vi "Read Instrument ID.vi"(8 "error in (no error)":errorcluster, 11 "Generic Instrument in":refnum<class "Generic Instrument.lvclass">) -> (0 "error out":errorcluster, 2 "Instrument ID":string, 3 "Generic Instrument out":refnum<class "Generic Instrument.lvclass">)   [LabVIEW 2014, in "Generic Instrument.lvlib" / "Generic Instrument.lvclass"]
uses:
  Generic Instrument.lvclass
  Generic Instrument.lvclass/Generic Instrument.ctl
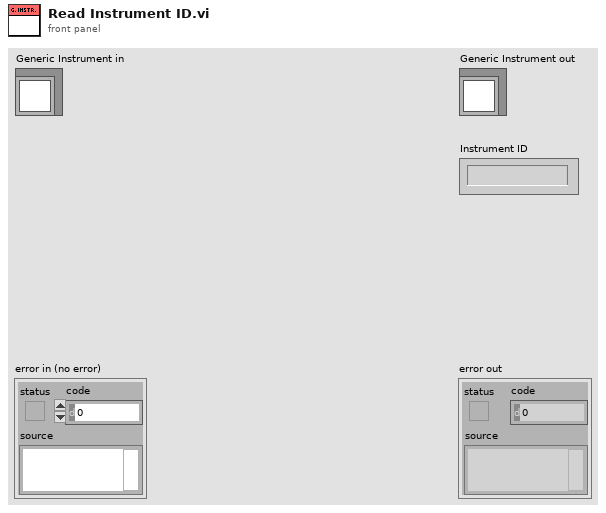
[diagram p1: front panel]
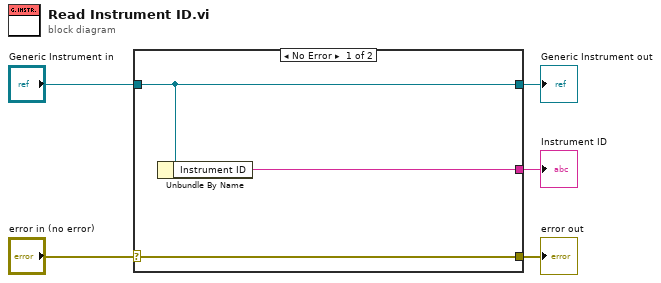
[diagram p0: block diagram]
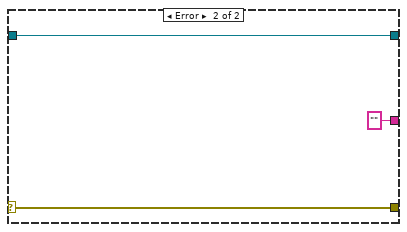
[diagram p2: hidden frame]
diagram:
  n1 = case shown="No Error" "error in (no error)" {
    selector: "error in (no error)" -> [w8 w10]
    tunnel: [w8 w10] -> w4
    tunnel: [w7 w11] -> w2
    tunnel: "Generic Instrument in" -> [w7 w11]
    tunnel: [w6 "" ("Instrument ID")] -> w1
    frame No Error {
      n2 = Unbundle By Name(w7) -> ("Instrument ID"=w6:string)
    }
    frame Error {
    }
  }
  "error out" <- w4
  "Generic Instrument out" <- w2
  "Instrument ID" <- w1
